vi "Test Map to Array - Map Elements.vi"(8 "error in":errorcluster) -> (0 "error out":errorcluster, 2 "passed":bool)   [LabVIEW 2020]
uses:
  2183a770-0473-3fdd-803c-8aeb4b9cb93f.vi
  source/library/Map to VArray of Clusters.vi
  source/library/Get Collection Subtype.vi
  source/library/Array of Clusters to VMap.vi
  <vilib>/addons/_JKI Toolkits/Caraya/classes/Assert/Assert True.vi
  <vilib>/addons/_JKI Toolkits/Caraya/classes/Test/Test.lvclass
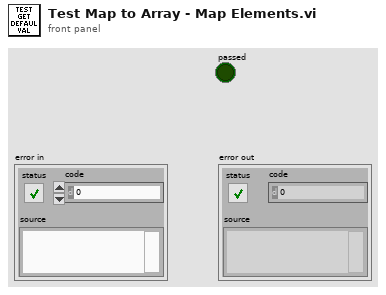
[diagram p1: front panel]
types:
  T1 = map{string, map{string, cluster{"key":string, "value":i32}}}
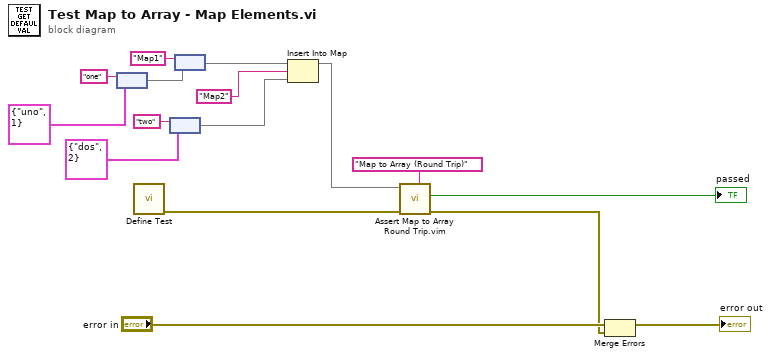
[diagram p0: block diagram]
diagram:
  n1 = node("one" ("key"), cluster{"key":string, "value":i32} {"key"="uno", "value"=1}) -> (w8:map{string, cluster{"key":string, "value":i32}})
  n2 = call <vilib>:"Define Test.vi"() -> ("error out"=w12:errorcluster)  [unwired: 11 in]
  n3 = node("two" ("key"), cluster{"key":string, "value":i32} {"key"="dos", "value"=2}) -> (w2:map{string, cluster{"key":string, "value":i32}})
  n4 = node("Map1" ("key"), w8) -> (w4:T1)
  n5 = Insert Into Map(map in=w4, key="Map2", value=w2) -> (map out=w1:T1)  [unwired: 2 out]
  n6 = call "Assert Map to Array Round Trip.vim"("Label"="Map to Array (Round Trip)", "error in (no error)"=w12, "Map"=w1) -> ("error out"=w14:errorcluster, "Passed"=→"passed":bool)  [unwired: 7 in]
  n7 = Merge Errors("error in", w14) -> (→"error out":errorcluster)
